vi "Input_Sensors_Turret.vi"(8 "Camera Hozinontal Angle Offset":dbl, 9 "Found Target":bool=TRUE) -> (3 "Turret Sensor Inputs":T1)   [LabVIEW 2012]
uses:
  Inputs_Sensors_Turret.ctl
  <vilib>/Rock Robotics/WPI/CAN/Jaguar/SubVIs/WPI_CANJaguar_StatusSelect.ctl
panel:
  out "error out":errorcluster
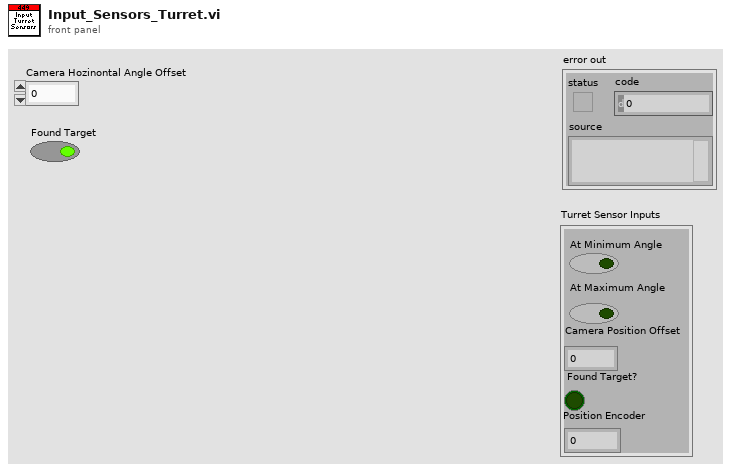
[diagram p1: front panel]
types:
  T1 = typedef "Inputs_Sensors_Turret.ctl" = cluster{"At Minimum Angle":bool, "At Maximum Angle":bool, "Camera Position Offset":dbl, "Found Target?":bool, "Position Encoder":dbl}
  T2 = typedef "WPI_CANJaguar_StatusSelect.ctl" = enum16{"Output Percent VBus", "Output Voltage", "Bus Voltage", "Current", "Temperature", "Position", "Speed", "Limit Switches", "Faults", "Fault Counters", "Power Cycle"}
  T3 = typedef "WPI_MotorControlDeviceRef.ctl" = cluster{"DeviceStatus":errorcluster, "Type":enum16{"PWM", "CAN"}, "PWM":cluster{"Digital Module":T4, "PWM Channel":T5, "DeadBand":T6}, "CAN":cluster{"Device Number":u8, "Control Mode":T7, "Semaphore":T8, "Max Vout":dbl}, "Invert":bool, "TransformRef":T9, "InvTransformRef":T9}
  T4 = typedef "FPGA_TypedefDigitalModule.ctl" = enum16{"Digital Module 1", "Digital Module 2"}
  T5 = typedef "FPGA_DIOPWMChannel.ctl" = enum8{"PWM 1", "PWM 2", "PWM 3", "PWM 4", "PWM 5", "PWM 6", "PWM 7", "PWM 8", "PWM 9", "PWM 10", "Invalid"}
  T6 = typedef "WPI_PWMDeadband.ctl" = cluster{"Name":string, "maxPositivePwm":i32, "minPositivePwm":i32, "centerPwm":i32, "maxNegativePwm":i32, "minNegativePwm":i32, "angularRange":u16}
  T7 = typedef "WPI_CANJaguar_ControlMode.ctl" = enum8{"Percent VBus", "Current", "Speed", "Position", "Voltage"}
  T8 = typedef "Semaphore RefNum" = refnum<k1>
  T9 = typedef "WPI_PWMTransform_ConPane.ctl" = refnum<vi>
  T10 = typedef "WPI_CANJaguar_Status.ctl" = cluster{"Output Percent VBus":dbl, "Output Voltage":dbl, "Bus Voltage":dbl, "Current":dbl, "Temperature":dbl, "Position":dbl, "Speed":dbl, "Limits":cluster{"Forward Limit":bool, "Reverse Limit":bool, "Forward Soft Limit":bool, "Reverse Soft Limit":bool, "Sticky Forward Limit":bool, "Sticky Reverse Limit":bool, "Sticky Forward Soft Limit":bool, "Sticky Reverse Soft Limit":bool}, "Faults":cluster{"Current Fault":bool, "Temperature Fault":bool, "Bus Voltage Fault":bool, "Gate Driver Fault":bool, "Comm Fault":bool}, "Fault Counters":cluster{"Current Faults":u8, "Temperature Faults":u8, "Bus Voltage Faults":u8, "Gate Driver Faults":u8, "Comm Faults":u8, "CAN Status":u8, "CAN RX Errors":u8, "CAN TX Errors":u8}, "Power Cycle":bool}
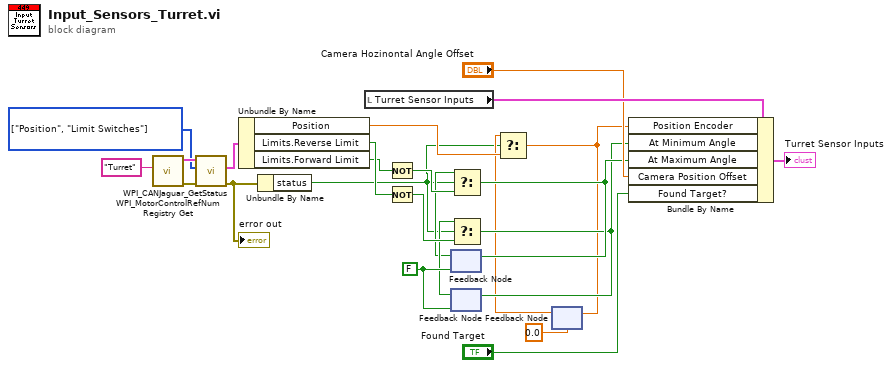
[diagram p0: block diagram]
diagram:
  w12 = FALSE
  w19 = T2[] [enum."Position", enum."Limit Switches"] items=["Output Percent VBus", "Output Voltage", "Bus Voltage", "Current", "Temperature", "Position", "Speed", "Limit Switches", "Faults", "Fault Counters", "Power Cycle"] ("Status Select")
  n1 = call <vilib>:"WPI_MotorControlRefNum Registry Get.vi"("refnum name"="Turret") -> ("error out"=w21:errorcluster, "MotorControlDevRef"=w20:T3)  [unwired: 9 in]
  n2 = call <vilib>:"WPI_CANJaguar_GetStatus.vi"("error in (no error)"=w21, "Status Select"=w19, "CAN Jaguar Ref"=w20) -> ("error out"=w13:errorcluster, "Status"=w18:T10)  [unwired: 6 in, 1 out]
  "error out" <- w13
  n3 = Unbundle By Name(w18) -> ("Position"=w3:dbl, "Limits.Reverse Limit"=w17:bool, "Limits.Forward Limit"=w15:bool)
  n4 = Unbundle By Name(w13) -> ("status"=w1:bool)
  n5 = local read "Turret Sensor Inputs"() -> (w24:T1)
  n6 = Not(x=w15) -> (.not. x?=w8:bool)
  n7 = Not(x=w17) -> (.not. x?=w9:bool)
  n8 = feedback #1(w12) -> (w6:bool)
  n9 = feedback #2(w12) -> (w7:bool)
  n10 = Select(t=w6, s=w1, f=w8) -> (s? t:f=w11:bool)
  n11 = feedback-in #1(w11) -> ()
  n12 = Select(t=w7, s=w1, f=w9) -> (s? t:f=w10:bool)
  n13 = feedback-in #2(w10) -> ()
  n14 = feedback #3(0.0 ("Position")) -> (w2:dbl)
  n15 = Select(t=w2, s=w1, f=w3) -> (s? t:f=w4:dbl)
  n16 = feedback-in #3(w4) -> ()
  n17 = Bundle By Name(cluster=w24, "Position Encoder"=w4, "At Minimum Angle"=w10, "At Maximum Angle"=w11, "Camera Position Offset"="Camera Hozinontal Angle Offset", "Found Target?"="Found Target") -> (→"Turret Sensor Inputs":T1)
